vi "RSZVB Channel Add Trace.vi"(5 "Channel (1)":i32=1, 6 "Trace Name (Trc1)":string="Trc1", 7 "Channel Name (Ch1)":string="Ch1", 8 "error in (no error)":errorcluster {"code" format="%.0x"}, 9 "Window (Trace) (1)":i32=1, 10 "Window (1)":i32=1, 11 "VISA session":refnum<visa-resource-name>) -> (0 "error out":errorcluster {"code" format="%.0x"}, 3 "dup VISA session":refnum<visa-resource-name>)   [LabVIEW 2011]
doc: "This VI creates a new channel and a new trace, which is displayed in the selected existing diagram area. The new channel settings (including a possible channel calibration) is preset to the default settings; the trace is created with the default trace settings.\n\nRemote-control command(s):\nCONFigure:CHANnel<Ch>[:STATe] ON\nCONFigure:CHANnel<Ch>:NAME '<string>'\nCALCulate<Ch>:PARameter:SDEFine '<string>', 'S21'\nDISPlay:WINDow<Wnd>:TRACe<WndTr>:FEED '<string>'"
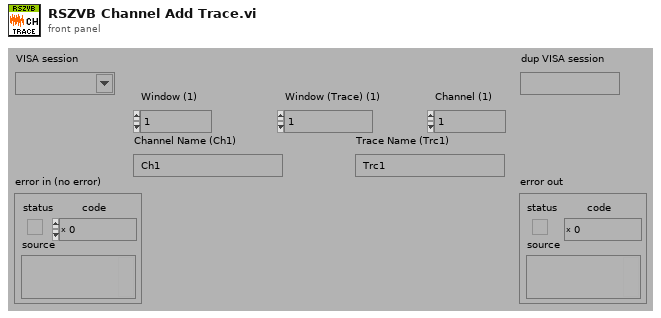
[diagram p1: front panel]
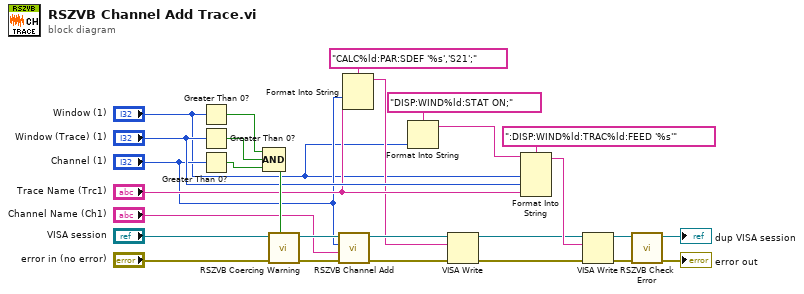
[diagram p0: block diagram]
diagram:
  n1 = Greater Than 0?(x="Window (1)") -> (x > 0?=w19:bool)
  n2 = Greater Than 0?(x="Window (Trace) (1)") -> (x > 0?=w18:bool)
  n3 = Greater Than 0?(x="Channel (1)") -> (x > 0?=w17:bool)
  n4 = Compound Arithmetic op=AND(w19, w18, w17) -> (w24:bool)
  n5 = call "RSZVB Coercing Warning.vi"("In Range?"=w24, "error in (no error)"="error in (no error)", "VISA session"="VISA session") -> ("error out"=w11:errorcluster, "dup VISA session"=w12:refnum<visa-resource-name>)  [unwired: 7 in]
  n6 = call "RSZVB Channel Add.vi"("error in (no error)"=w11, "Channel Name (Ch1)"="Channel Name (Ch1)", "Channel (1)"="Channel (1)", "VISA session"=w12) -> ("error out"=w6:errorcluster, "dup VISA session"=w7:refnum<visa-resource-name>)  [unwired: 6 in]
  n7 = Format Into String(format string="CALC%ld:PAR:SDEF '%s','S21';", "Channel (1)", "Trace Name (Trc1)") -> (resulting string=w3:string)  [unwired: 2 in, 1 out]
  n8 = Format Into String(format string="DISP:WIND%ld:STAT ON;", "Window (1)") -> (resulting string=w2:string)  [unwired: 2 in, 1 out]
  n9 = VISA Write(VISA resource name=w7, write buffer=w3, error in (no error)=w6) -> (VISA resource name out=w4:refnum<visa-resource-name>, error out=w5:errorcluster)  [unwired: 1 out]
  n10 = Format Into String(format string=":DISP:WIND%ld:TRAC%ld:FEED '%s'", initial string=w2, "Window (1)", "Window (Trace) (1)", "Trace Name (Trc1)") -> (resulting string=w14:string)  [unwired: 1 in, 1 out]
  n11 = VISA Write(VISA resource name=w4, write buffer=w14, error in (no error)=w5) -> (VISA resource name out=w25:refnum<visa-resource-name>, error out=w26:errorcluster)  [unwired: 1 out]
  n12 = call "RSZVB Check Error.vi"("error in (no error)"=w26, "VISA session"=w25) -> ("error out"=→"error out":errorcluster, "dup VISA session"=→"dup VISA session":refnum<visa-resource-name>)  [unwired: 8 in]
